vi "DisplayQuick.vi"(8 "error in (no error)":errorcluster, 11 "DisplayTetrodes in":refnum<class "DisplayTetrodes.lvclass">) -> (0 "error out":errorcluster)   [LabVIEW 2010, in "DisplayTetrodes.lvclass"]
uses:
  DisplayTetrodes.lvclass
  <vilib>/Analysis/3filter.llb/Butterworth Filter (DBL).vi
  Program Files/National Instruments/LabVIEW 2010/resource/objmgr/ni.dex.rc
  <vilib>/Analysis/NI_AALBase.lvlib
panel:
  out "Numeric 2":i32
  in  "DisplayTime (sec)":dbl(slide) scale=0.0..5.0
  in  "FilterData":bool
  in  "Low Cutoff":dbl=50.0 format="%0.4f"
  in  "High Cutoff":dbl=500.0 format="%0.2f"
  out "Connected":bool
  out "Waveform Chart":dbl[][](graph)
  in  "STOP":bool
  out "Numeric":i32
  in  "Scale":dbl=1.6934e-10
  in  "Spacing":dbl=0.002
  out "Elements in stream":i32(slide) scale=0.0..100.0
  in  "Network Stream Writer IP":string(combo)
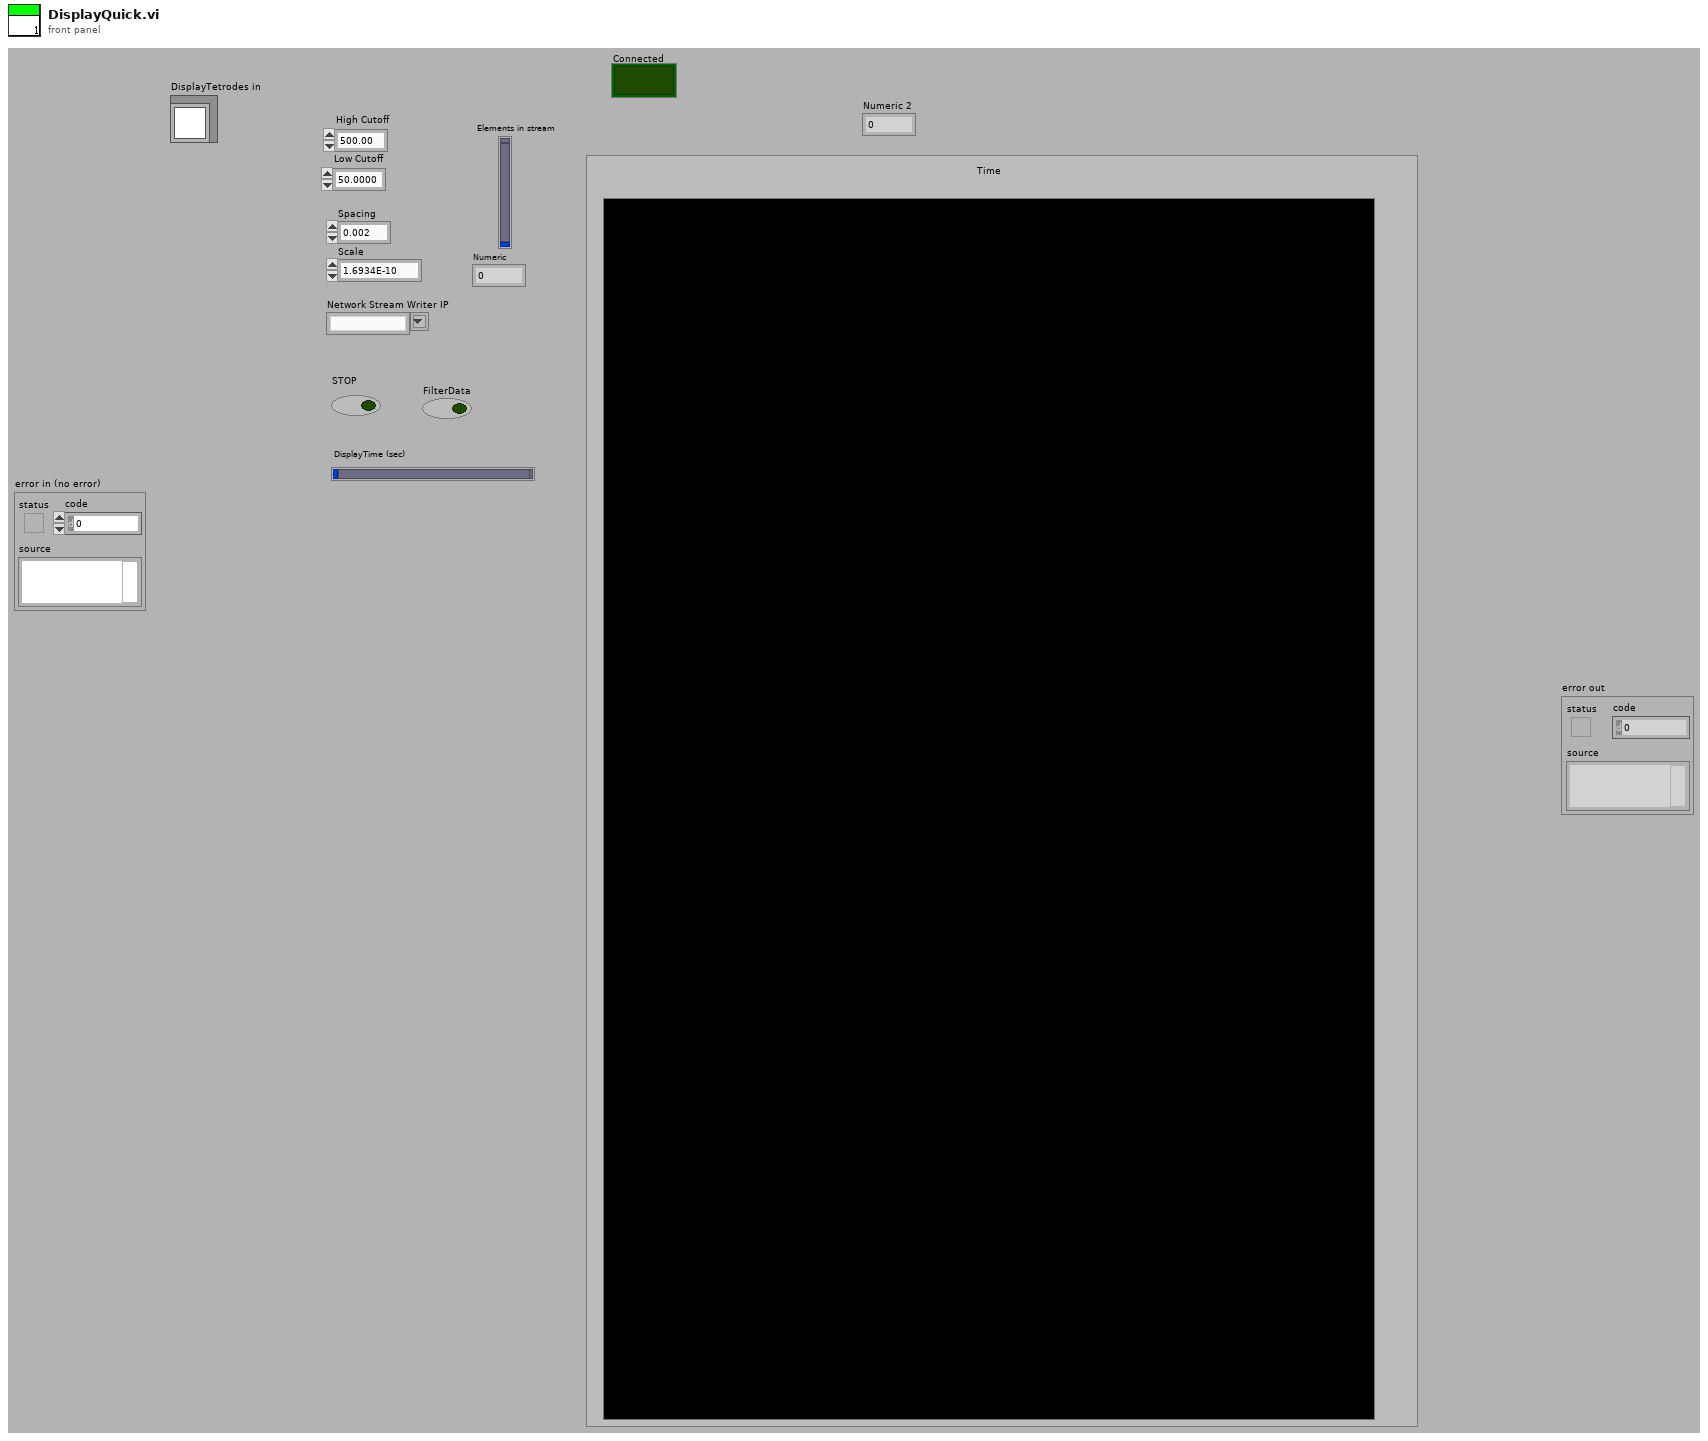
[diagram p1: front panel]
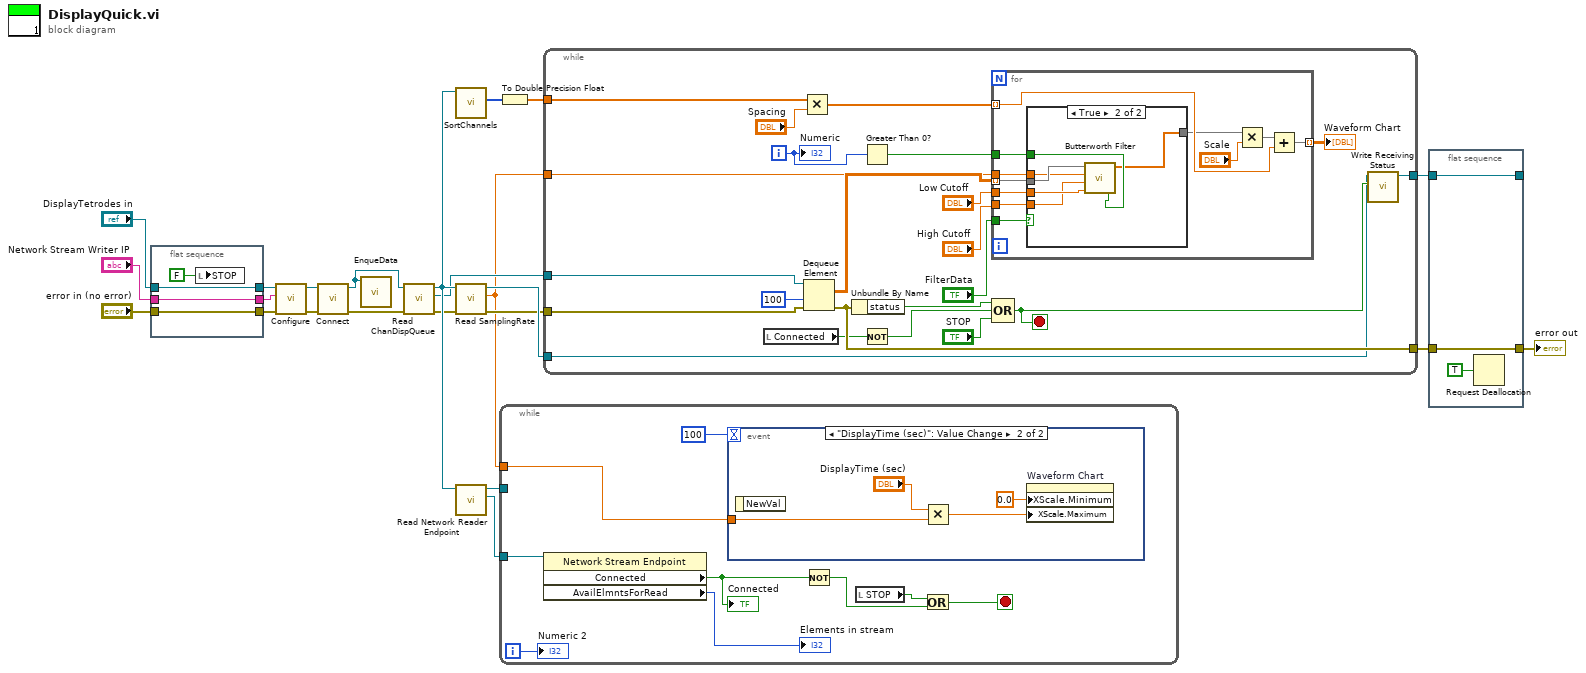
[diagram p0: block diagram]
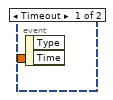
[diagram p2: hidden frame]
diagram:
  n1 = flat-sequence {
    tunnel: "DisplayTetrodes in" -> [w27]
    tunnel: [w27] -> w11
    tunnel: "Network Stream Writer IP" -> [w26]
    tunnel: [w26] -> w9
    tunnel: "error in (no error)" -> [w25]
    tunnel: [w25] -> w7
    frame #0 {
      n2 = local write "STOP"(FALSE ("STOP")) -> ()
    }
  }
  n3 = call-dynamic "Configure.vi"("error in (no error)"=w7, "Network Stream Writer IP"=w9, "DataReceiver in"=w11) -> ("error out"=w17:errorcluster, "DataReceiver out"=w19:refnum<class "DisplayTetrodes.lvclass">)  [unwired: 7 in]
  n4 = call-dynamic "Connect.vi"("error in (no error)"=w17, "DataReceiver in"=w19) -> ("error out"=w16:errorcluster, "DataReceiver out"=w18:refnum<class "DisplayTetrodes.lvclass">)  [unwired: 8 in]
  n5 = call-dynamic "EnqueData.vi"("DataReceiver in"=w18) -> ()  [unwired: 9 in, 2 out]
  n6 = call-dynamic "Read ChanDispQueue.vi"("error in (no error)"=w16, "DataReceiver in"=w18) -> ("error out"=w20:errorcluster, "ChanDispQueue"=w21:refnum<queue>, "DataReceiver out"=w22:refnum<class "DisplayTetrodes.lvclass">)  [unwired: 7 in]
  n7 = call-dynamic "SortChannels.vi"("DisplayTetrodes in"=w22) -> ("reorderedChanNums"=w6:i32[])  [unwired: 3 in, 7 out]
  n8 = call-dynamic "Read SamplingRate.vi"("error in (no error)"=w20, "DataReceiver in"=w22) -> ("error out"=w2:errorcluster, "SamplingRate"=w1:dbl, "DataReceiver out"=w3:refnum<class "DisplayTetrodes.lvclass">)  [unwired: 7 in]
  n9 = call-dynamic "Read Network Reader Endpoint.vi"("DataReceiver in"=w22) -> ("Network Stream Reader Endpoint"=w23:refnum<k21>, "DataReceiver out"=w4:refnum<class "DisplayTetrodes.lvclass">)  [unwired: 8 in, 1 out]
  n10 = To Double Precision Float(number=w6) -> (double precision float=w5:dbl[])
  n11 = while {
    tunnel: w23 -> [w36]
    tunnel: w4 -> [_]
    tunnel: w1 -> [w29]
    i -> [w28]
    stop <- w34 stop-if-true
    n12 = property class="Network Stream Endpoint"(reference=w36) -> ("Connected"=w31:bool, "AvailElmntsForRead"=→"Elements in stream":i32)  [unwired: 1 in, 2 out]
    "Connected" <- w31
    n13 = event shown="[1] \"DisplayTime (sec)\": Value Change" {
      selector: _ -> [_ _]
      dyn-events: _ -> [_ _]
      timeout: u32 100 ("millisecond multiple") -> [_ _]
      tunnel: w29 -> [_ w37]
      event Timeout {
        n14 = event-data() -> ()  [unwired: 1 in, 2 out]
      }
      event "DisplayTime (sec)": Value Change {
        n15 = event-data() -> ()  [unwired: 1 in, 1 out]
        n16 = Multiply(x="DisplayTime (sec)", y=w37) -> (x*y=w39:dbl)
        n17 = property on="Waveform Chart" class="WFChart (strict)"("XScale.Minimum"=0.0 ("X Scale.Range:Minimum"), "XScale.Maximum"=w39) -> ()  [unwired: 2 in, 2 out]
      }
    }
    n18 = Not(x=w31) -> (.not. x?=w32:bool)
    n19 = local read "STOP"() -> (w33:bool)
    n20 = Or(x=w33, y=w32) -> (x .or. y?=w34:bool)
    "Numeric 2" <- w28
  }
  n21 = while {
    tunnel: [w54] -> w15
    tunnel: w21 -> [w57]
    tunnel: w3 -> [w42]
    tunnel: [w55] -> w13
    tunnel: w5 -> [w51]
    tunnel: w2 -> [w49]
    tunnel: w1 -> [w41]
    i -> [w61]
    stop <- w56 stop-if-true
    n22 = local read "Connected"() -> (w52:bool)
    n23 = Multiply(x=w51, y="Spacing") -> (x*y=w58:dbl[])
    n24 = Dequeue Element(queue=w57, timeout in ms (-1)=100, error in (no error)=w49) -> (element=w62:dbl[][], error out=w54:errorcluster)  [unwired: 2 out]
    n25 = Unbundle By Name(w54) -> ("status"=w46:bool)
    n26 = Greater Than 0?(x=w61) -> (x > 0?=w60:bool)
    n27 = Not(x=w52) -> (.not. x?=w47:bool)
    n28 = for {
      tunnel: w62 -> [w70] mode=indexing
      tunnel: w60 -> [w68]
      tunnel: w58 -> [w72] mode=indexing
      tunnel: [w71] -> w50 mode=indexing
      tunnel: "FilterData" -> [w67]
      tunnel: "High Cutoff" -> [w65]
      tunnel: "Low Cutoff" -> [w64]
      tunnel: w41 -> [w63]
      n29 = case shown="True" w67 {
        tunnel: w70 -> [w74 w80]
        tunnel: [w74 w75] -> w69
        tunnel: w68 -> [_ w76]
        tunnel: w65 -> [_ w78]
        tunnel: w64 -> [_ w79]
        tunnel: w63 -> [_ w77]
        frame False {
        }
        frame True {
          n30 = call-poly <vilib>:"Butterworth Filter.vi"("init/cont (init:F)"=w76, "low cutoff freq: fl"=w79, "high cutoff freq: fh"=w78, "sampling freq: fs"=w77, "X"=w80) -> ("Filtered X"=w75:dbl[])  [unwired: 3 in, 1 out]
        }
      }
      n31 = Multiply(x=w69, y="Scale") -> (x*y=w73:dbl[])
      n32 = Add(x=w73, y=w72) -> (x+y=w71:dbl[])
    }
    "Waveform Chart" <- w50
    n33 = Compound Arithmetic op=OR(w46, w47, "STOP") -> (w56:bool)
    n34 = call-dynamic "Write Receiving Status.vi"("Stop Reading"=w56, "DataReceiver in"=w42) -> ("DataReceiver out"=w55:refnum<class "DisplayTetrodes.lvclass">)  [unwired: 8 in, 1 out]
    "Numeric" <- w61
  }
  n35 = flat-sequence {
    tunnel: w15 -> [w82]
    tunnel: [w82] -> w14
    tunnel: w13 -> [w81]
    tunnel: [w81] -> _
    frame #0 {
      n36 = Request Deallocation(TRUE ("flag")) -> ()
    }
  }
  "error out" <- w14
